vi "Sequence Data to Sytem CMDs.vi"(11 "Sequence Data":T12 {"Traverse"."Angle" scale format="%.3f"; "Traverse"."Velocity" scale=-1.0..1.0 scale format="%.1f"; "Auto Angle" scale format="%.3f"}) -> (1 "CMD Intake":T1, 2 "CMD_ACT_Drive_Data Out":T5 {"Auto Angle" scale format="%.3f"; "Direction"."Rotate(Yaw) CCW 1 CW -1" scale=1.0..-1.0; "Direction"."Traverse"."Angle" scale format="%.3f"; "Direction"."Traverse"."Velocity" scale=-1.0..1.0 scale format="%.1f"}, 3 "CMD_ACT_shooter_Data":T3, 5 "Max Wait Time Out":dbl)   [LabVIEW 2023, in "2023-Auto_CMD.lvlib"]
uses:
  2023-Auto_CMD.lvlib
  Shared Code/TypeDefs/Cluster_Auto Sequence Settings.ctl
  ENUM_Drive Mode Select.ctl
  Shared Code/TypeDefs/Dial_Compase heading unit circle CCW positive.ctl
  Shared Code/TypeDefs/Cluster_Module Velocity-Direction-Rotations.ctl
  Shared Code/TypeDefs/Level_Velocity plus-minus 1.ctl
  SwerveDrive/Cluster_CMD_ACT_Data.ctl
  Shared Code/TypeDefs/ENUM_CMD_Mode Select.ctl
  Shared Code/TypeDefs/Cluster_CMD_Direction Data.ctl
  Shared Code/TypeDefs/Cluster_X-Y.ctl
  Shooter/Cluster_CMD_ACT_Data.ctl
  Shooter/ENUM_Shooter_Mode.ctl
  2024 Intake/Cluster_CMD_ACT_Data.ctl
  2024 Intake/ENUM_Shooter_Mode.ctl
  SwerveDrive/SwerveDrive_ACT_ts.lvlib
  Shooter/Shooter_ACT.lvlib
  2024 Intake/Intake_ACT.lvlib
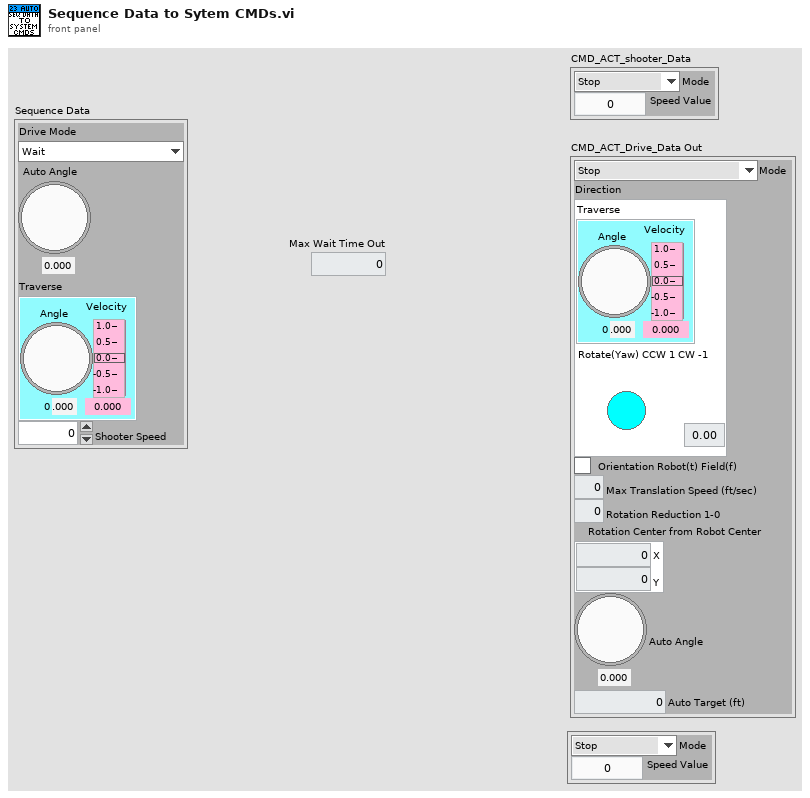
[diagram p1: front panel]
types:
  T1 = typedef "Intake_ACT.lvlib/Cluster_CMD_ACT_Data.ctl" = cluster{"Mode":T2, "Speed Value":dbl}
  T2 = typedef "Intake_ACT.lvlib/ENUM_Shooter_Mode.ctl" = enum16{"Stop", "Speed Percent", "Speed RPM"}
  T3 = typedef "Shooter_ACT.lvlib/Cluster_CMD_ACT_Data.ctl" = cluster{"Mode":T4, "Speed Value":dbl}
  T4 = typedef "Shooter_ACT.lvlib/ENUM_Shooter_Mode.ctl" = enum16{"Stop", "Speed Percent", "Speed RPM", "AutoShoot"}
  T5 = typedef "SwerveDrive_ACT_ts.lvlib/Cluster_CMD_ACT_Data.ctl" = cluster{"Mode":T6, "Direction":T7, "Orientation Robot(t) Field(f)":bool, "Max Translation Speed (ft/sec)":dbl, "Rotation Reduction 1-0":dbl, "Rotation Center from Robot Center":T11, "Auto Angle":T10, "Auto Target (ft)":dbl}
  T6 = typedef "ENUM_CMD_Mode Select.ctl" = enum16{"Stop", "Translate Cmd Rotate Cmd", "Translate Cmd Rotate Auto"}
  T7 = typedef "Cluster_CMD_Direction Data.ctl" = cluster{"Traverse":T8, "Rotate(Yaw) CCW 1 CW -1":dbl}
  T8 = typedef "Cluster_Module Velocity-Direction-Rotations.ctl" = cluster{"Velocity":T9, "Angle":T10, "Rotations Count":dbl}
  T9 = typedef "Level_Velocity plus-minus 1.ctl" = dbl
  T10 = typedef "Dial_Compase heading unit circle CCW positive.ctl" = dbl
  T11 = typedef "Cluster_X-Y.ctl" = cluster{"X":dbl, "Y":dbl}
  T12 = typedef "Cluster_Auto Sequence Settings.ctl" = cluster{"Drive Mode":T13, "Auto Angle":T10, "Traverse":T8, "Shooter Speed":dbl}
  T13 = typedef "2023-Auto_CMD.lvlib/ENUM_Drive Mode Select.ctl" = enum16{"Wait", "Timed Direction Drive", "Rotate to Angle", "Stop", "Auto Shoot"}
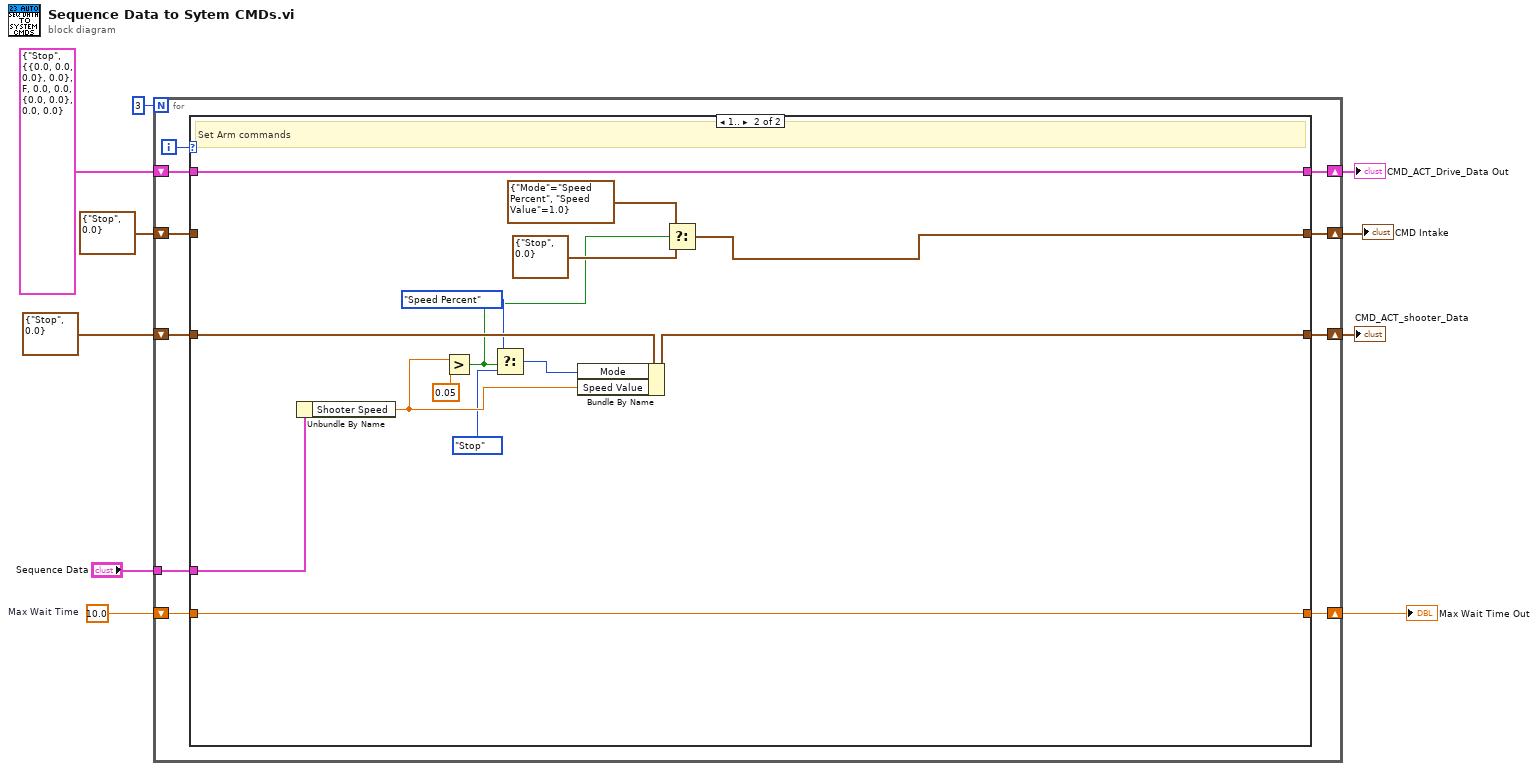
[diagram p0: block diagram]
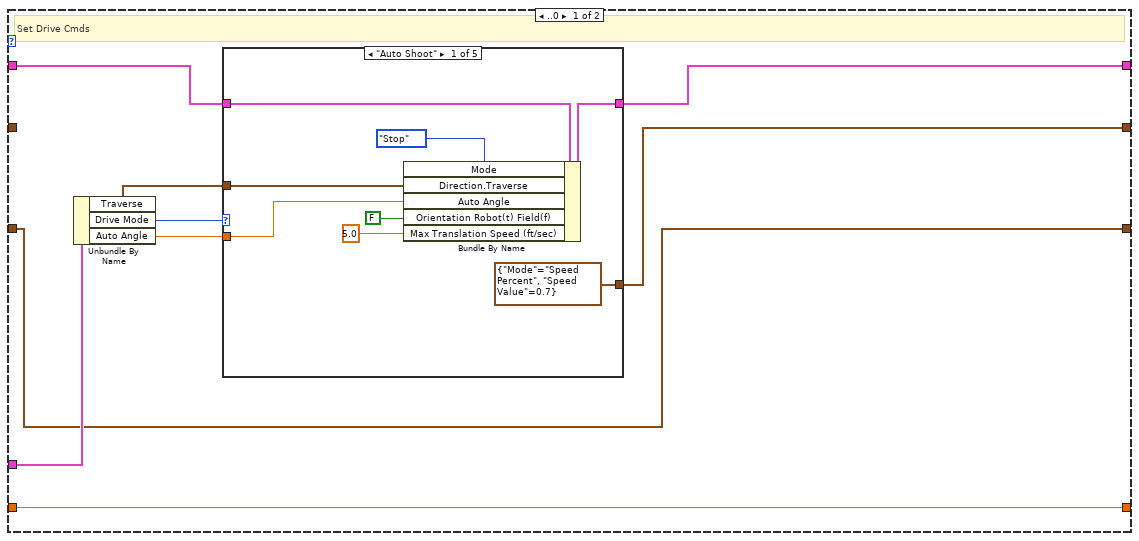
[diagram p2: hidden frame]
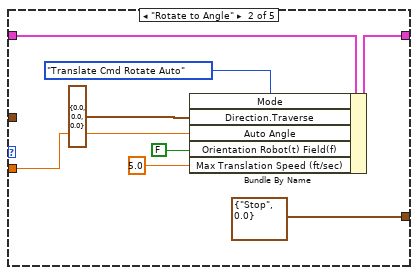
[diagram p3: hidden frame]
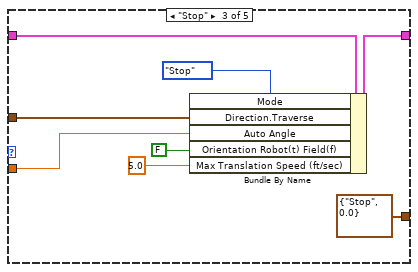
[diagram p4: hidden frame]
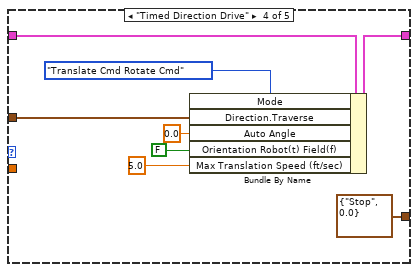
[diagram p5: hidden frame]
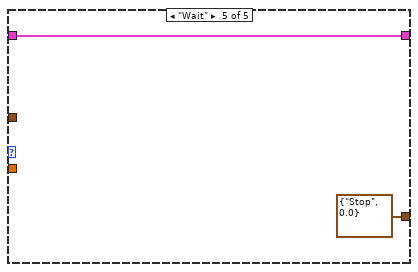
[diagram p6: hidden frame]
diagram:
  w9 = 10.0  # Max Wait Time
  n1 = for {
    N: 3 -> [_]
    tunnel: "Sequence Data" -> [w17]
    shift-right: [w18] -> w5
    shift-left: T5 {"Mode"=enum."Stop", "Direction"={"Traverse"={"Velocity"=0.0, "Angle"=0.0, "Rotations Count"=0.0}, "Rotate(Yaw) CCW 1 CW -1"=0.0}, "Orientation Robot(t) Field(f)"=FALSE, "Max Translation Speed (ft/sec)"=0.0, "Rotation Reduction 1-0"=0.0, "Rotation Center from Robot Center"={"X"=0.0, "Y"=0.0}, "Auto Angle"=0.0, "Auto Target (ft)"=0.0} ("CMD_ACT_Drive_Data Out") -> [w19]
    shift-right: [w15] -> w8
    shift-left: w9 -> [w16]
    shift-right: [w13] -> w3
    shift-left: T3 {"Mode"=enum."Stop", "Speed Value"=0.0} ("CMD_ACT_Template_Data") -> [w14]
    shift-right: [w11] -> w2
    shift-left: T1 {"Mode"=enum."Stop", "Speed Value"=0.0} ("CMD Intake") -> [w12]
    i -> [w20]
    n2 = case shown="1.." w20 {
      tunnel: w19 -> [w25 w77]
      tunnel: [w24 w77] -> w18
      tunnel: w17 -> [w28 w76]
      tunnel: w16 -> [w29 w73]
      tunnel: [w29 w73] -> w15
      tunnel: w14 -> [w22 w75]
      tunnel: [w22 w74] -> w13
      tunnel: w12 -> [_ _]
      tunnel: [w21 w65] -> w11
      frame ..0 {
        # "Set Drive Cmds"
        n3 = Unbundle By Name(w28) -> ("Traverse"=w23:T8, "Drive Mode"=w27:T13, "Auto Angle"=w26:T10)
        n4 = case shown="\"Auto Shoot\"" w27 {
          tunnel: w26 -> [w31 w40 w47 _ _]
          tunnel: w25 -> [w36 w44 w52 w60 w63]
          tunnel: [w35 w43 w51 w59 w63] -> w24
          tunnel: w23 -> [w32 _ w48 w56 _]
          tunnel: [T1 {"Mode"=enum."Speed Percent", "Speed Value"=0.7} ("CMD Intake") T1 {"Mode"=enum."Stop", "Speed Value"=0.0} ("CMD Intake") T1 {"Mode"=enum."Stop", "Speed Value"=0.0} ("CMD Intake") T1 {"Mode"=enum."Stop", "Speed Value"=0.0} ("CMD Intake") T1 {"Mode"=enum."Stop", "Speed Value"=0.0} ("CMD Intake")] -> w21
          frame "Auto Shoot" {
            n5 = Bundle By Name(cluster=w36, "Mode"=ENUM_CMD_Mode_Select."Stop", "Direction.Traverse"=w32, "Auto Angle"=w31, "Orientation Robot(t) Field(f)"=FALSE, "Max Translation Speed (ft/sec)"=5.0) -> (w35:T5)
          }
          frame "Rotate to Angle" {
            n6 = Bundle By Name(cluster=w44, "Mode"=ENUM_CMD_Mode_Select."Translate Cmd Rotate Auto", "Direction.Traverse"=T8 {"Velocity"=0.0, "Angle"=0.0, "Rotations Count"=0.0}, "Auto Angle"=w40, "Orientation Robot(t) Field(f)"=FALSE, "Max Translation Speed (ft/sec)"=5.0) -> (w43:T5)
          }
          frame "Stop" {
            n7 = Bundle By Name(cluster=w52, "Mode"=ENUM_CMD_Mode_Select."Stop", "Direction.Traverse"=w48, "Auto Angle"=w47, "Orientation Robot(t) Field(f)"=FALSE, "Max Translation Speed (ft/sec)"=5.0) -> (w51:T5)
          }
          frame "Timed Direction Drive" {
            n8 = Bundle By Name(cluster=w60, "Mode"=ENUM_CMD_Mode_Select."Translate Cmd Rotate Cmd", "Direction.Traverse"=w56, "Auto Angle"=T10 0.0, "Orientation Robot(t) Field(f)"=FALSE, "Max Translation Speed (ft/sec)"=5.0) -> (w59:T5)
          }
          frame "Wait" {
          }
        }
      }
      frame 1.. {
        # "Set Arm commands"
        n9 = Unbundle By Name(w76) -> ("Shooter Speed"=w72:dbl)
        n10 = Greater?(x=w72, y=0.05) -> (0:w64:bool)
        n11 = Select(t=ENUM_Shooter_Mode."Speed Percent" ("Mode"), s=w64, f=ENUM_Shooter_Mode."Stop" ("Mode")) -> (s? t:f=w69:T4)
        n12 = Bundle By Name(cluster=w75, "Mode"=w69, "Speed Value"=w72) -> (w74:T3)
        n13 = Select(t=T1 {"Mode"=enum."Speed Percent", "Speed Value"=1.0} ("CMD Intake"), s=w64, f=T1 {"Mode"=enum."Stop", "Speed Value"=0.0} ("CMD Intake")) -> (s? t:f=w65:T1)
      }
    }
  }
  "Max Wait Time Out" <- w8
  "CMD_ACT_Drive_Data Out" <- w5
  "CMD_ACT_shooter_Data" <- w3
  "CMD Intake" <- w2
